vi "staticUpdate.vi"(8 "error in (no error)":errorcluster, 10 "staticChannelUpdate":T1, 11 "AtomChipHWC in":refnum<class "AtomChipHWC.lvclass">) -> (0 "error out":errorcluster, 3 "AtomChipHWC out":refnum<class "AtomChipHWC.lvclass">)   [LabVIEW 2011, in "Hardware.lvlib" / "HWControllers.lvlib" / "AtomChipHWC.lvclass"]
doc: "Update the output state of a channel to a new value"
uses:
  AtomChipHWC.lvclass
  AtomChipHWC.lvclass/AtomChipHWC.ctl
  Channels/Digital/DigitalOutput.lvclass
  Channels/VoltOutput/AnalogOutput.lvclass
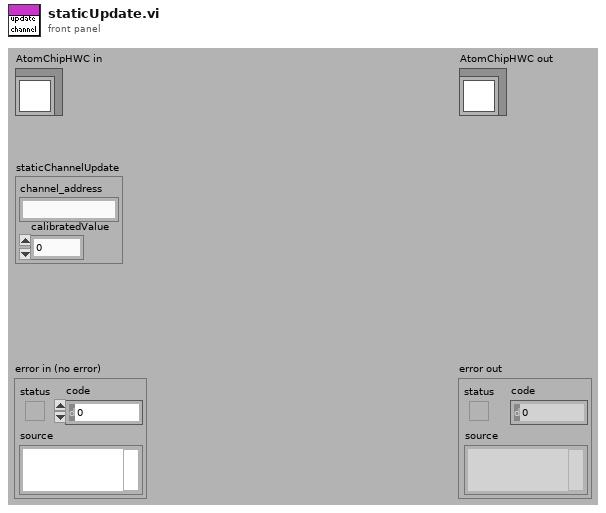
[diagram p1: front panel]
types:
  T1 = cluster{"channel_address":string, "calibratedValue":dbl}
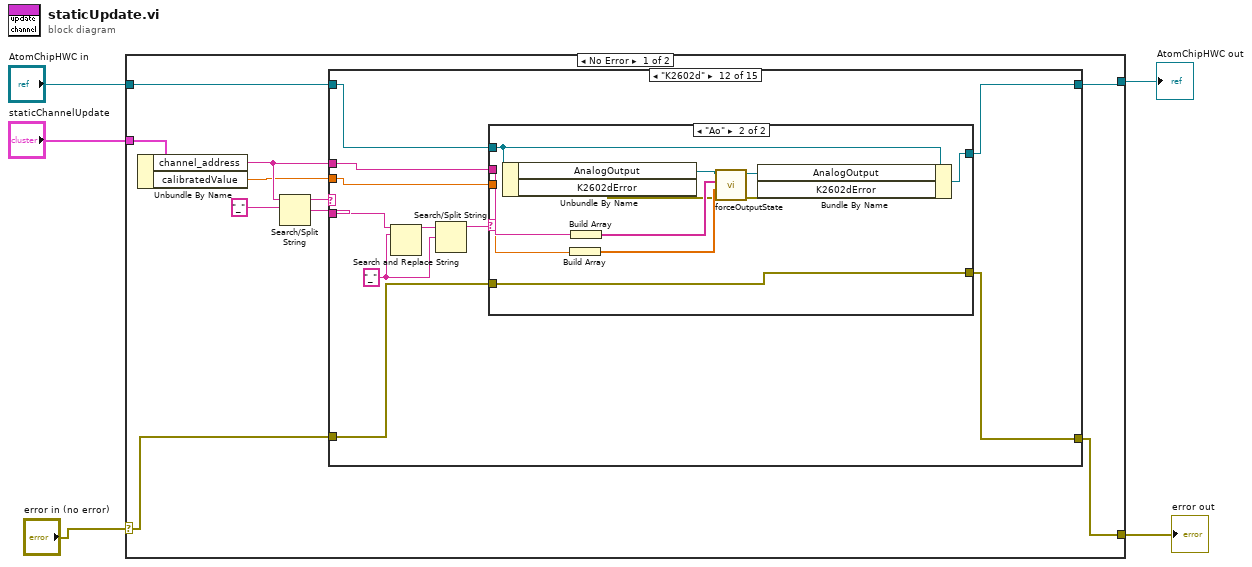
[diagram p0: block diagram]
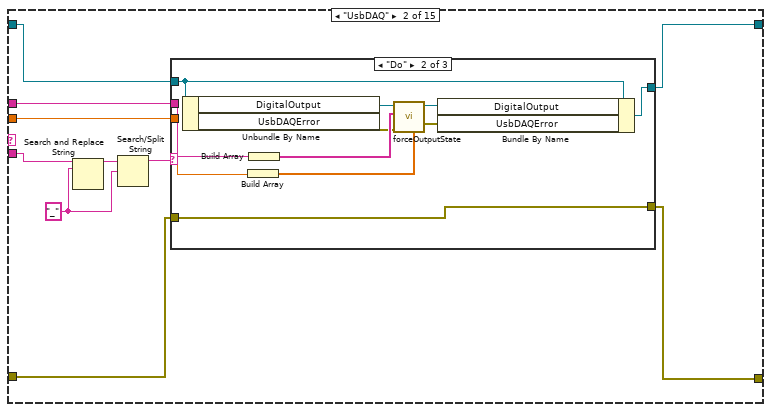
[diagram p3: hidden frame]
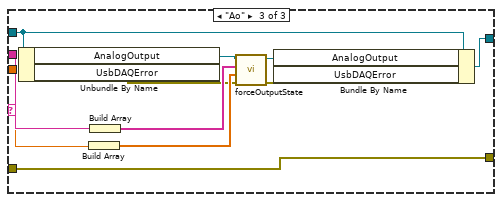
[diagram p5: hidden frame]
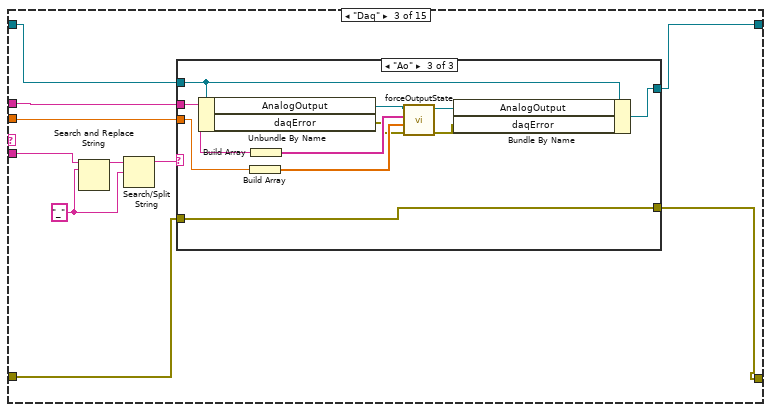
[diagram p6: hidden frame]
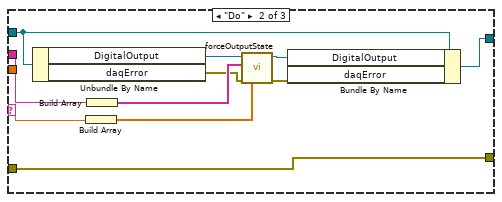
[diagram p8: hidden frame]
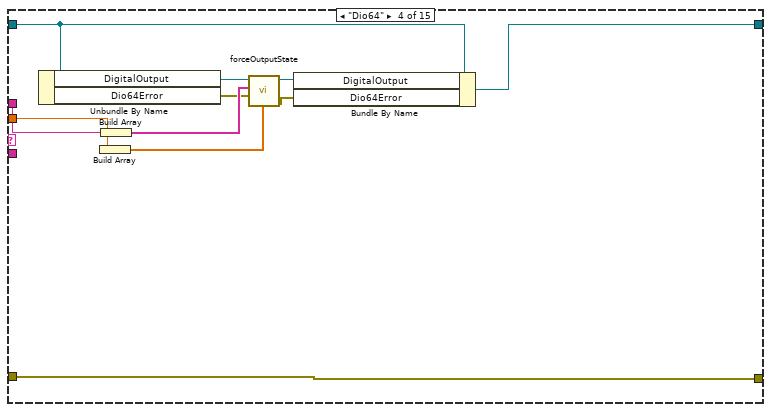
[diagram p9: hidden frame]
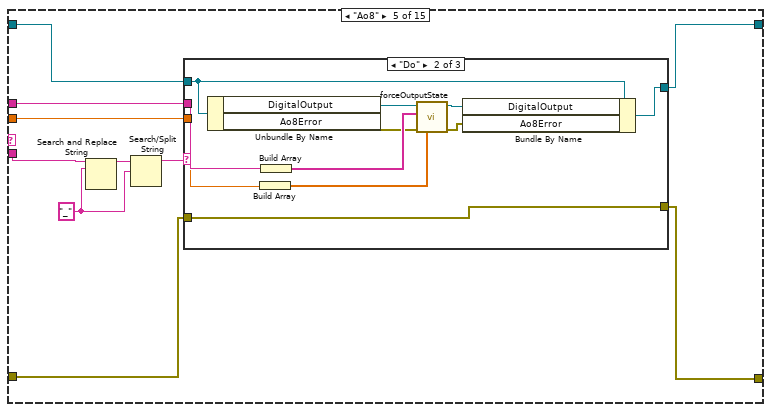
[diagram p10: hidden frame]
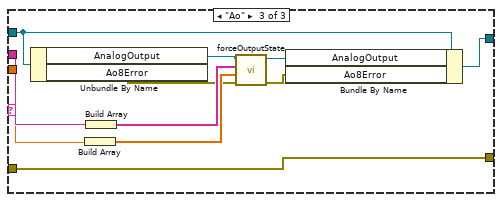
[diagram p12: hidden frame]
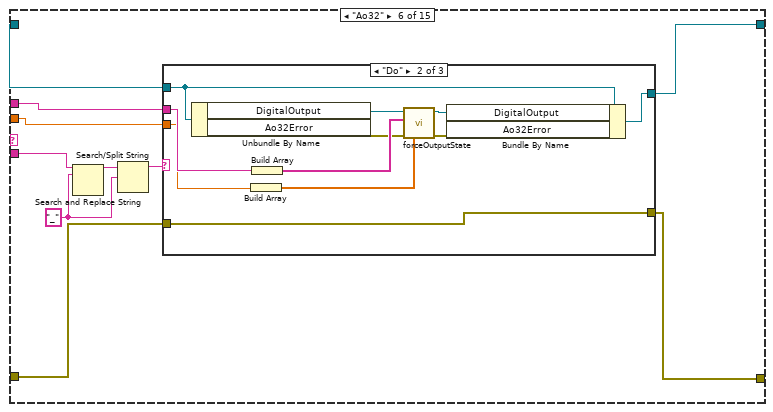
[diagram p13: hidden frame]
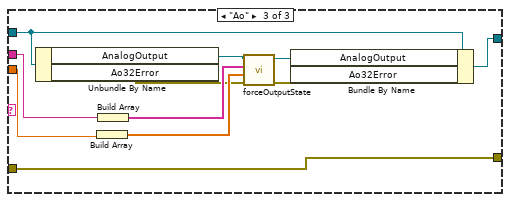
[diagram p15: hidden frame]
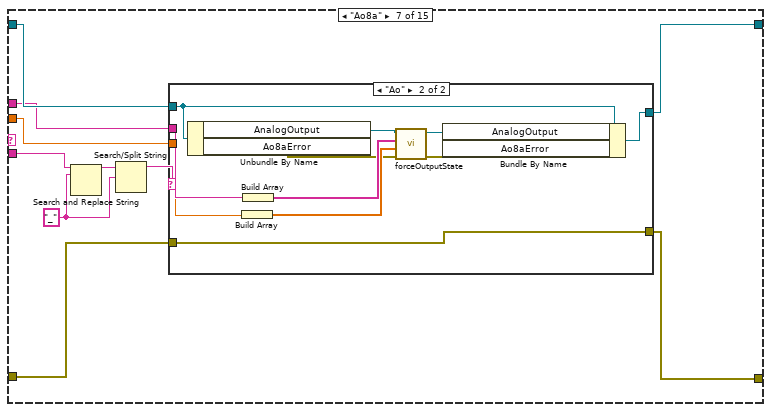
[diagram p16: hidden frame]
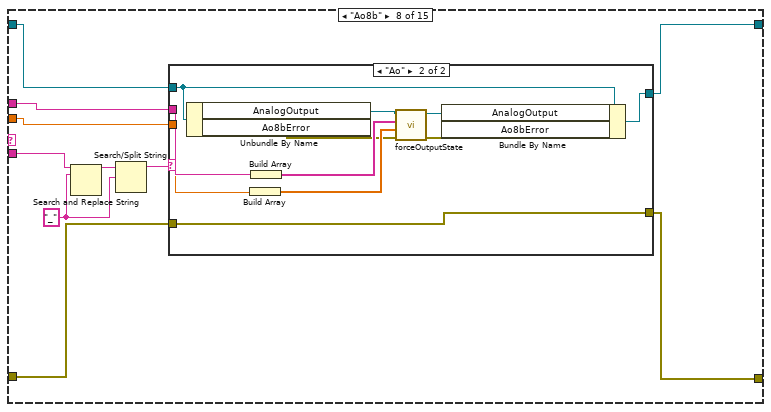
[diagram p18: hidden frame]
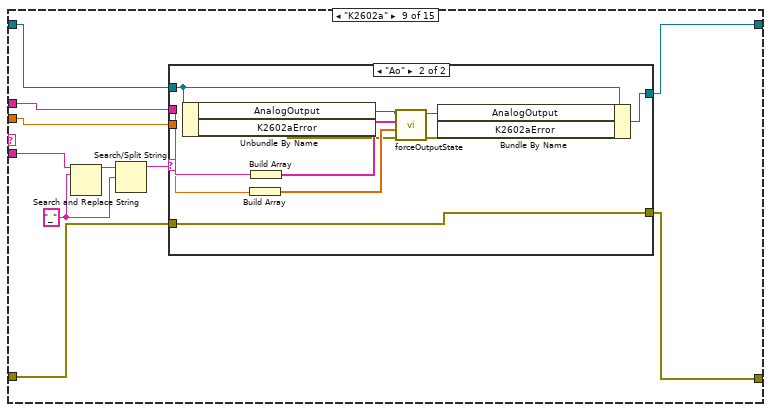
[diagram p20: hidden frame]
diagram:
  n1 = case shown="No Error" "error in (no error)" {
    selector: "error in (no error)" -> [w9 w336]
    tunnel: [w8 w336] -> w4
    tunnel: [w10 w337] -> w1
    tunnel: "AtomChipHWC in" -> [w11 w337]
    tunnel: "staticChannelUpdate" -> [w15 _]
    frame No Error {
      n2 = Unbundle By Name(w15) -> ("channel_address"=w12:string, "calibratedValue"=w7:dbl)
      n3 = Search/Split String(string=w12, search string/char (-)="_") -> (substring before match=w13:string, match + rest of string=w6:string)  [unwired: 1 in, 1 out]
      n4 = case shown="\"K2602d\"" w13 {
        tunnel: w12 -> [_ w24 w58 w95 w105 w134 w168 w191 w214 w237 w260 w283 w311 w322 w333]
        tunnel: w11 -> [w17 w21 w55 w92 w106 w137 w171 w194 w217 w240 w263 w286 w313 w324 w335]
        tunnel: [w17 w20 w54 w90 w99 w136 w170 w193 w216 w239 w262 w285 w312 w323 w334] -> w10
        tunnel: w9 -> [w16 w19 w52 w86 w98 w132 w166 w189 w212 w235 w258 w281 w309 w320 w331]
        tunnel: [w16 w18 w53 w86 w97 w131 w165 w188 w211 w234 w257 w280 w309 w320 w331] -> w8
        tunnel: w7 -> [_ w23 w57 w89 w104 w133 w167 w190 w213 w236 w259 w282 w310 w321 w332]
        tunnel: w6 -> [_ w22 w56 _ w103 w135 w169 w192 w215 w238 w261 w284 _ _ _]
        frame "No Hardware", Default {
        }
        frame "UsbDAQ" {
          w26 = "_"
          n5 = Search and Replace String(input string=w22, search string=w26) -> (result string=w27:string)  [unwired: 6 in, 3 out]
          n6 = Search/Split String(string=w27, search string/char (-)=w26) -> (substring before match=w25:string)  [unwired: 1 in, 2 out]
          n7 = case shown="\"Do\"" w25 {
            tunnel: w21 -> [w29 w34 w49]
            tunnel: w24 -> [_ w36 w51]
            tunnel: w23 -> [_ w35 w50]
            tunnel: [w29 w33 w48] -> w20
            tunnel: w19 -> [w28 w30 w41]
            tunnel: [w28 w30 w41] -> w18
            frame Default {
            }
            frame "Do" {
              n8 = Unbundle By Name(w34) -> ("DigitalOutput"=w40:refnum<class "DigitalOutput.lvclass">, "UsbDAQError"=w32:errorcluster)
              n9 = Build Array(w35) -> (w38:dbl[])
              n10 = Build Array(w36) -> (w39:string[])
              n11 = call-dynamic "forceOutputState.vi"("error in (no error)"=w32, "calibratedValues"=w38, "channel_addresses"=w39, "DigitalOutput in"=w40) -> ("error out"=w31:errorcluster, "DigitalOutput out"=w37:refnum<class "DigitalOutput.lvclass">)  [unwired: 6 in]
              n12 = Bundle By Name(cluster=w34, "DigitalOutput"=w37, "UsbDAQError"=w31) -> (w33:refnum<class "AtomChipHWC.lvclass">)
            }
            frame "Ao" {
              n13 = Unbundle By Name(w49) -> ("AnalogOutput"=w47:refnum<class "AnalogOutput.lvclass">, "UsbDAQError"=w43:errorcluster)
              n14 = Build Array(w50) -> (w44:dbl[])
              n15 = Build Array(w51) -> (w45:string[])
              n16 = call-dynamic "forceOutputState.vi"("error in (no error)"=w43, "calibratedValues"=w44, "channel_addresses"=w45, "AnalogOutput in"=w47) -> ("error out"=w42:errorcluster, "AnalogOutput out"=w46:refnum<class "AnalogOutput.lvclass">)  [unwired: 6 in]
              n17 = Bundle By Name(cluster=w49, "AnalogOutput"=w46, "UsbDAQError"=w42) -> (w48:refnum<class "AtomChipHWC.lvclass">)
            }
          }
        }
        frame "Daq" {
          w60 = "_"
          n18 = Search and Replace String(input string=w56, search string=w60) -> (result string=w61:string)  [unwired: 6 in, 3 out]
          n19 = Search/Split String(string=w61, search string/char (-)=w60) -> (substring before match=w59:string)  [unwired: 1 in, 2 out]
          n20 = case shown="\"Ao\"" w59 {
            tunnel: w55 -> [w63 w68 w83]
            tunnel: w58 -> [_ w70 w85]
            tunnel: w57 -> [_ w69 w84]
            tunnel: [w63 w67 w82] -> w54
            tunnel: w52 -> [w62 w65 w76]
            tunnel: [w62 w65 w76] -> w53
            frame Default {
            }
            frame "Do" {
              n21 = Unbundle By Name(w68) -> ("DigitalOutput"=w74:refnum<class "DigitalOutput.lvclass">, "daqError"=w66:errorcluster)
              n22 = Build Array(w69) -> (w72:dbl[])
              n23 = Build Array(w70) -> (w73:string[])
              n24 = call-dynamic "forceOutputState.vi"("error in (no error)"=w66, "calibratedValues"=w72, "channel_addresses"=w73, "DigitalOutput in"=w74) -> ("error out"=w64:errorcluster, "DigitalOutput out"=w71:refnum<class "DigitalOutput.lvclass">)  [unwired: 6 in]
              n25 = Bundle By Name(cluster=w68, "DigitalOutput"=w71, "daqError"=w64) -> (w67:refnum<class "AtomChipHWC.lvclass">)
            }
            frame "Ao" {
              n26 = Unbundle By Name(w83) -> ("AnalogOutput"=w81:refnum<class "AnalogOutput.lvclass">, "daqError"=w77:errorcluster)
              n27 = Build Array(w84) -> (w78:dbl[])
              n28 = Build Array(w85) -> (w79:string[])
              n29 = call-dynamic "forceOutputState.vi"("error in (no error)"=w77, "calibratedValues"=w78, "channel_addresses"=w79, "AnalogOutput in"=w81) -> ("error out"=w75:errorcluster, "AnalogOutput out"=w80:refnum<class "AnalogOutput.lvclass">)  [unwired: 6 in]
              n30 = Bundle By Name(cluster=w83, "AnalogOutput"=w80, "daqError"=w75) -> (w82:refnum<class "AtomChipHWC.lvclass">)
            }
          }
        }
        frame "Dio64" {
          n31 = Unbundle By Name(w92) -> ("DigitalOutput"=w96:refnum<class "DigitalOutput.lvclass">, "Dio64Error"=w88:errorcluster)
          n32 = Build Array(w89) -> (w93:dbl[])
          n33 = Build Array(w95) -> (w94:string[])
          n34 = call-dynamic "forceOutputState.vi"("error in (no error)"=w88, "calibratedValues"=w93, "channel_addresses"=w94, "DigitalOutput in"=w96) -> ("error out"=w87:errorcluster, "DigitalOutput out"=w91:refnum<class "DigitalOutput.lvclass">)  [unwired: 6 in]
          n35 = Bundle By Name(cluster=w92, "DigitalOutput"=w91, "Dio64Error"=w87) -> (w90:refnum<class "AtomChipHWC.lvclass">)
        }
        frame "Ao8" {
          w101 = "_"
          n36 = Search and Replace String(input string=w103, search string=w101) -> (result string=w102:string)  [unwired: 6 in, 3 out]
          n37 = Search/Split String(string=w102, search string/char (-)=w101) -> (substring before match=w100:string)  [unwired: 1 in, 2 out]
          n38 = case shown="\"Do\"" w100 {
            tunnel: w106 -> [w108 w113 w128]
            tunnel: w105 -> [_ w115 w130]
            tunnel: w104 -> [_ w114 w129]
            tunnel: [w108 w112 w127] -> w99
            tunnel: w98 -> [w107 w109 w120]
            tunnel: [w107 w109 w120] -> w97
            frame Default {
            }
            frame "Do" {
              n39 = Unbundle By Name(w113) -> ("DigitalOutput"=w119:refnum<class "DigitalOutput.lvclass">, "Ao8Error"=w111:errorcluster)
              n40 = Build Array(w114) -> (w117:dbl[])
              n41 = Build Array(w115) -> (w118:string[])
              n42 = call-dynamic "forceOutputState.vi"("error in (no error)"=w111, "calibratedValues"=w117, "channel_addresses"=w118, "DigitalOutput in"=w119) -> ("error out"=w110:errorcluster, "DigitalOutput out"=w116:refnum<class "DigitalOutput.lvclass">)  [unwired: 6 in]
              n43 = Bundle By Name(cluster=w113, "DigitalOutput"=w116, "Ao8Error"=w110) -> (w112:refnum<class "AtomChipHWC.lvclass">)
            }
            frame "Ao" {
              n44 = Unbundle By Name(w128) -> ("AnalogOutput"=w126:refnum<class "AnalogOutput.lvclass">, "Ao8Error"=w122:errorcluster)
              n45 = Build Array(w129) -> (w123:dbl[])
              n46 = Build Array(w130) -> (w124:string[])
              n47 = call-dynamic "forceOutputState.vi"("error in (no error)"=w122, "calibratedValues"=w123, "channel_addresses"=w124, "AnalogOutput in"=w126) -> ("error out"=w121:errorcluster, "AnalogOutput out"=w125:refnum<class "AnalogOutput.lvclass">)  [unwired: 6 in]
              n48 = Bundle By Name(cluster=w128, "AnalogOutput"=w125, "Ao8Error"=w121) -> (w127:refnum<class "AtomChipHWC.lvclass">)
            }
          }
        }
        frame "Ao32" {
          w139 = "_"
          n49 = Search and Replace String(input string=w135, search string=w139) -> (result string=w140:string)  [unwired: 6 in, 3 out]
          n50 = Search/Split String(string=w140, search string/char (-)=w139) -> (substring before match=w138:string)  [unwired: 1 in, 2 out]
          n51 = case shown="\"Do\"" w138 {
            tunnel: w137 -> [w142 w147 w162]
            tunnel: w134 -> [_ w149 w164]
            tunnel: w133 -> [_ w148 w163]
            tunnel: [w142 w146 w161] -> w136
            tunnel: w132 -> [w141 w143 w154]
            tunnel: [w141 w143 w154] -> w131
            frame Default {
            }
            frame "Do" {
              n52 = Unbundle By Name(w147) -> ("DigitalOutput"=w153:refnum<class "DigitalOutput.lvclass">, "Ao32Error"=w145:errorcluster)
              n53 = Build Array(w148) -> (w151:dbl[])
              n54 = Build Array(w149) -> (w152:string[])
              n55 = call-dynamic "forceOutputState.vi"("error in (no error)"=w145, "calibratedValues"=w151, "channel_addresses"=w152, "DigitalOutput in"=w153) -> ("error out"=w144:errorcluster, "DigitalOutput out"=w150:refnum<class "DigitalOutput.lvclass">)  [unwired: 6 in]
              n56 = Bundle By Name(cluster=w147, "DigitalOutput"=w150, "Ao32Error"=w144) -> (w146:refnum<class "AtomChipHWC.lvclass">)
            }
            frame "Ao" {
              n57 = Unbundle By Name(w162) -> ("AnalogOutput"=w160:refnum<class "AnalogOutput.lvclass">, "Ao32Error"=w156:errorcluster)
              n58 = Build Array(w163) -> (w157:dbl[])
              n59 = Build Array(w164) -> (w158:string[])
              n60 = call-dynamic "forceOutputState.vi"("error in (no error)"=w156, "calibratedValues"=w157, "channel_addresses"=w158, "AnalogOutput in"=w160) -> ("error out"=w155:errorcluster, "AnalogOutput out"=w159:refnum<class "AnalogOutput.lvclass">)  [unwired: 6 in]
              n61 = Bundle By Name(cluster=w162, "AnalogOutput"=w159, "Ao32Error"=w155) -> (w161:refnum<class "AtomChipHWC.lvclass">)
            }
          }
        }
        frame "Ao8a" {
          w173 = "_"
          n62 = Search and Replace String(input string=w169, search string=w173) -> (result string=w174:string)  [unwired: 6 in, 3 out]
          n63 = Search/Split String(string=w174, search string/char (-)=w173) -> (substring before match=w172:string)  [unwired: 1 in, 2 out]
          n64 = case shown="\"Ao\"" w172 {
            tunnel: w171 -> [w176 w185]
            tunnel: w168 -> [_ w187]
            tunnel: w167 -> [_ w186]
            tunnel: [w176 w184] -> w170
            tunnel: w166 -> [w175 w177]
            tunnel: [w175 w177] -> w165
            frame Default {
            }
            frame "Ao" {
              n65 = Unbundle By Name(w185) -> ("AnalogOutput"=w183:refnum<class "AnalogOutput.lvclass">, "Ao8aError"=w179:errorcluster)
              n66 = Build Array(w186) -> (w180:dbl[])
              n67 = Build Array(w187) -> (w181:string[])
              n68 = call-dynamic "forceOutputState.vi"("error in (no error)"=w179, "calibratedValues"=w180, "channel_addresses"=w181, "AnalogOutput in"=w183) -> ("error out"=w178:errorcluster, "AnalogOutput out"=w182:refnum<class "AnalogOutput.lvclass">)  [unwired: 6 in]
              n69 = Bundle By Name(cluster=w185, "AnalogOutput"=w182, "Ao8aError"=w178) -> (w184:refnum<class "AtomChipHWC.lvclass">)
            }
          }
        }
        frame "Ao8b" {
          w196 = "_"
          n70 = Search and Replace String(input string=w192, search string=w196) -> (result string=w197:string)  [unwired: 6 in, 3 out]
          n71 = Search/Split String(string=w197, search string/char (-)=w196) -> (substring before match=w195:string)  [unwired: 1 in, 2 out]
          n72 = case shown="\"Ao\"" w195 {
            tunnel: w194 -> [w199 w208]
            tunnel: w191 -> [_ w210]
            tunnel: w190 -> [_ w209]
            tunnel: [w199 w207] -> w193
            tunnel: w189 -> [w198 w201]
            tunnel: [w198 w201] -> w188
            frame Default {
            }
            frame "Ao" {
              n73 = Unbundle By Name(w208) -> ("AnalogOutput"=w206:refnum<class "AnalogOutput.lvclass">, "Ao8bError"=w202:errorcluster)
              n74 = Build Array(w209) -> (w203:dbl[])
              n75 = Build Array(w210) -> (w204:string[])
              n76 = call-dynamic "forceOutputState.vi"("error in (no error)"=w202, "calibratedValues"=w203, "channel_addresses"=w204, "AnalogOutput in"=w206) -> ("error out"=w200:errorcluster, "AnalogOutput out"=w205:refnum<class "AnalogOutput.lvclass">)  [unwired: 6 in]
              n77 = Bundle By Name(cluster=w208, "AnalogOutput"=w205, "Ao8bError"=w200) -> (w207:refnum<class "AtomChipHWC.lvclass">)
            }
          }
        }
        frame "K2602a" {
          w219 = "_"
          n78 = Search and Replace String(input string=w215, search string=w219) -> (result string=w220:string)  [unwired: 6 in, 3 out]
          n79 = Search/Split String(string=w220, search string/char (-)=w219) -> (substring before match=w218:string)  [unwired: 1 in, 2 out]
          n80 = case shown="\"Ao\"" w218 {
            tunnel: w217 -> [w222 w231]
            tunnel: w214 -> [_ w233]
            tunnel: w213 -> [_ w232]
            tunnel: [w222 w230] -> w216
            tunnel: w212 -> [w221 w224]
            tunnel: [w221 w224] -> w211
            frame Default {
            }
            frame "Ao" {
              n81 = Unbundle By Name(w231) -> ("AnalogOutput"=w229:refnum<class "AnalogOutput.lvclass">, "K2602aError"=w225:errorcluster)
              n82 = Build Array(w232) -> (w226:dbl[])
              n83 = Build Array(w233) -> (w227:string[])
              n84 = call-dynamic "forceOutputState.vi"("error in (no error)"=w225, "calibratedValues"=w226, "channel_addresses"=w227, "AnalogOutput in"=w229) -> ("error out"=w223:errorcluster, "AnalogOutput out"=w228:refnum<class "AnalogOutput.lvclass">)  [unwired: 6 in]
              n85 = Bundle By Name(cluster=w231, "AnalogOutput"=w228, "K2602aError"=w223) -> (w230:refnum<class "AtomChipHWC.lvclass">)
            }
          }
        }
        frame "K2602b" {
          w242 = "_"
          n86 = Search and Replace String(input string=w238, search string=w242) -> (result string=w243:string)  [unwired: 6 in, 3 out]
          n87 = Search/Split String(string=w243, search string/char (-)=w242) -> (substring before match=w241:string)  [unwired: 1 in, 2 out]
          n88 = case shown="\"Ao\"" w241 {
            tunnel: w240 -> [w245 w254]
            tunnel: w237 -> [_ w256]
            tunnel: w236 -> [_ w255]
            tunnel: [w245 w253] -> w239
            tunnel: w235 -> [w244 w247]
            tunnel: [w244 w247] -> w234
            frame Default {
            }
            frame "Ao" {
              n89 = Unbundle By Name(w254) -> ("AnalogOutput"=w252:refnum<class "AnalogOutput.lvclass">, "K2602bError"=w248:errorcluster)
              n90 = Build Array(w255) -> (w249:dbl[])
              n91 = Build Array(w256) -> (w250:string[])
              n92 = call-dynamic "forceOutputState.vi"("error in (no error)"=w248, "calibratedValues"=w249, "channel_addresses"=w250, "AnalogOutput in"=w252) -> ("error out"=w246:errorcluster, "AnalogOutput out"=w251:refnum<class "AnalogOutput.lvclass">)  [unwired: 6 in]
              n93 = Bundle By Name(cluster=w254, "AnalogOutput"=w251, "K2602bError"=w246) -> (w253:refnum<class "AtomChipHWC.lvclass">)
            }
          }
        }
        frame "K2602c" {
          w265 = "_"
          n94 = Search and Replace String(input string=w261, search string=w265) -> (result string=w266:string)  [unwired: 6 in, 3 out]
          n95 = Search/Split String(string=w266, search string/char (-)=w265) -> (substring before match=w264:string)  [unwired: 1 in, 2 out]
          n96 = case shown="\"Ao\"" w264 {
            tunnel: w263 -> [w268 w277]
            tunnel: w260 -> [_ w279]
            tunnel: w259 -> [_ w278]
            tunnel: [w268 w276] -> w262
            tunnel: w258 -> [w267 w270]
            tunnel: [w267 w270] -> w257
            frame Default {
            }
            frame "Ao" {
              n97 = Unbundle By Name(w277) -> ("AnalogOutput"=w275:refnum<class "AnalogOutput.lvclass">, "K2602cError"=w271:errorcluster)
              n98 = Build Array(w278) -> (w272:dbl[])
              n99 = Build Array(w279) -> (w273:string[])
              n100 = call-dynamic "forceOutputState.vi"("error in (no error)"=w271, "calibratedValues"=w272, "channel_addresses"=w273, "AnalogOutput in"=w275) -> ("error out"=w269:errorcluster, "AnalogOutput out"=w274:refnum<class "AnalogOutput.lvclass">)  [unwired: 6 in]
              n101 = Bundle By Name(cluster=w277, "AnalogOutput"=w274, "K2602cError"=w269) -> (w276:refnum<class "AtomChipHWC.lvclass">)
            }
          }
        }
        frame "K2602d" {
          w288 = "_"
          n102 = Search and Replace String(input string=w284, search string=w288) -> (result string=w289:string)  [unwired: 6 in, 3 out]
          n103 = Search/Split String(string=w289, search string/char (-)=w288) -> (substring before match=w287:string)  [unwired: 1 in, 2 out]
          n104 = case shown="\"Ao\"" w287 {
            tunnel: w286 -> [w291 w300]
            tunnel: w283 -> [_ w302]
            tunnel: w282 -> [_ w301]
            tunnel: [w291 w299] -> w285
            tunnel: w281 -> [w290 w293]
            tunnel: [w290 w293] -> w280
            frame Default {
            }
            frame "Ao" {
              n105 = Unbundle By Name(w300) -> ("AnalogOutput"=w298:refnum<class "AnalogOutput.lvclass">, "K2602dError"=w294:errorcluster)
              n106 = Build Array(w301) -> (w295:dbl[])
              n107 = Build Array(w302) -> (w296:string[])
              n108 = call-dynamic "forceOutputState.vi"("error in (no error)"=w294, "calibratedValues"=w295, "channel_addresses"=w296, "AnalogOutput in"=w298) -> ("error out"=w292:errorcluster, "AnalogOutput out"=w297:refnum<class "AnalogOutput.lvclass">)  [unwired: 6 in]
              n109 = Bundle By Name(cluster=w300, "AnalogOutput"=w297, "K2602dError"=w292) -> (w299:refnum<class "AtomChipHWC.lvclass">)
            }
          }
        }
        frame "HMP2020" {
          n110 = Unbundle By Name(w313) -> ("AnalogOutput"=w308:refnum<class "AnalogOutput.lvclass">, "2020Error"=w304:errorcluster)
          n111 = Build Array(w310) -> (w305:dbl[])
          n112 = Build Array(w311) -> (w306:string[])
          n113 = call-dynamic "forceOutputState.vi"("error in (no error)"=w304, "calibratedValues"=w305, "channel_addresses"=w306, "AnalogOutput in"=w308) -> ("error out"=w303:errorcluster, "AnalogOutput out"=w307:refnum<class "AnalogOutput.lvclass">)  [unwired: 6 in]
          n114 = Bundle By Name(cluster=w313, "AnalogOutput"=w307, "2020Error"=w303) -> (w312:refnum<class "AtomChipHWC.lvclass">)
        }
        frame "HMP2030" {
          n115 = Unbundle By Name(w324) -> ("AnalogOutput"=w319:refnum<class "AnalogOutput.lvclass">, "2030Error"=w315:errorcluster)
          n116 = Build Array(w321) -> (w316:dbl[])
          n117 = Build Array(w322) -> (w317:string[])
          n118 = call-dynamic "forceOutputState.vi"("error in (no error)"=w315, "calibratedValues"=w316, "channel_addresses"=w317, "AnalogOutput in"=w319) -> ("error out"=w314:errorcluster, "AnalogOutput out"=w318:refnum<class "AnalogOutput.lvclass">)  [unwired: 6 in]
          n119 = Bundle By Name(cluster=w324, "AnalogOutput"=w318, "2030Error"=w314) -> (w323:refnum<class "AtomChipHWC.lvclass">)
        }
        frame "HMP4030" {
          n120 = Unbundle By Name(w335) -> ("AnalogOutput"=w330:refnum<class "AnalogOutput.lvclass">, "4030Error"=w326:errorcluster)
          n121 = Build Array(w332) -> (w327:dbl[])
          n122 = Build Array(w333) -> (w328:string[])
          n123 = call-dynamic "forceOutputState.vi"("error in (no error)"=w326, "calibratedValues"=w327, "channel_addresses"=w328, "AnalogOutput in"=w330) -> ("error out"=w325:errorcluster, "AnalogOutput out"=w329:refnum<class "AnalogOutput.lvclass">)  [unwired: 6 in]
          n124 = Bundle By Name(cluster=w335, "AnalogOutput"=w329, "4030Error"=w325) -> (w334:refnum<class "AtomChipHWC.lvclass">)
        }
      }
    }
    frame Error {
    }
  }
  "error out" <- w4
  "AtomChipHWC out" <- w1
